vi "Disconnect.vi"(8 "error in (no error)":errorcluster, 11 "PalmSens in":refnum<class "PalmSens.lvclass">) -> (0 "error out":errorcluster, 3 "PalmSens out":refnum<class "PalmSens.lvclass">)   [LabVIEW 2020, in "PalmSens.lvclass"]
uses:
  PalmSens.lvclass
  PalmSens.lvclass/PalmSens.ctl
  C:/Utils/LabVIEWNETSDK - Class/PalmSens/Libraries/PalmSens.Core.Simplified.LabVIEW.dll
  Libraries/PalmSens.Core.Simplified.LabVIEW.dll
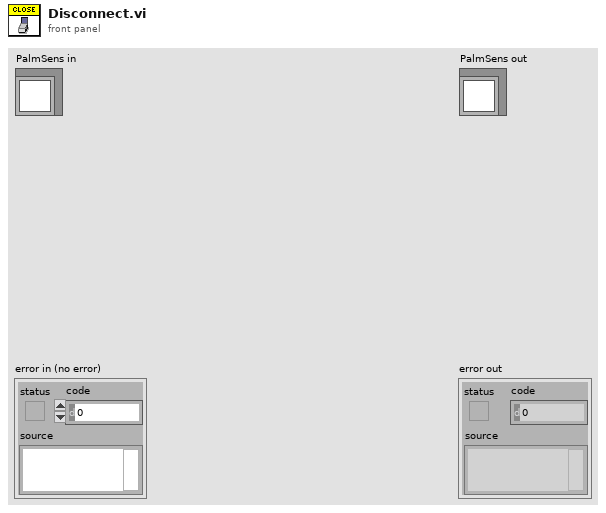
[diagram p1: front panel]
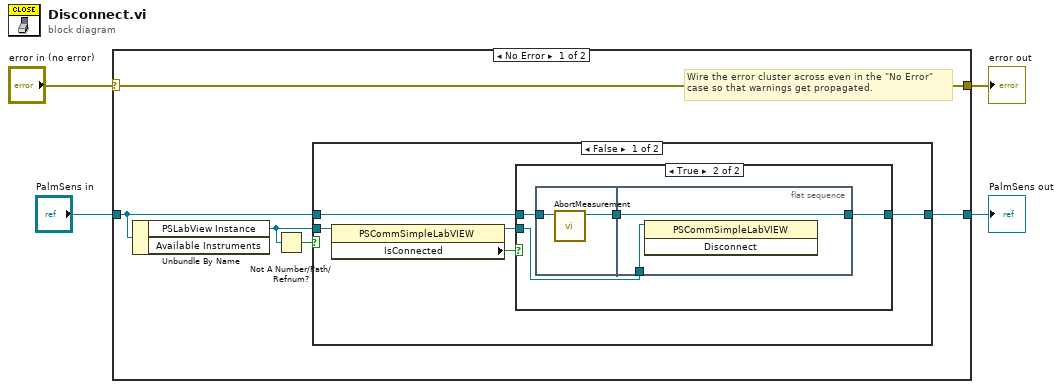
[diagram p0: block diagram]
diagram:
  n1 = case shown="No Error" "error in (no error)" {
    selector: "error in (no error)" -> [w9 w26]
    tunnel: [w9 w26] -> w3
    tunnel: [w5 w25] -> w1
    tunnel: "PalmSens in" -> [w6 w25]
    frame No Error {
      # "Wire the error cluster across even in the \"No Error\"\ncase so that warnings get propagated."
      n2 = Unbundle By Name(w6) -> ("PSLabView Instance"=w7:refnum<k24>)  [unwired: 1 out]
      n3 = Not A Number/Path/Refnum?(number/path/refnum=w7) -> (NaN/Path/Refnum?=w8:bool)
      n4 = case shown="False" w8 {
        tunnel: w7 -> [w14 _]
        tunnel: w6 -> [w11 w24]
        tunnel: [w10 w24] -> w5
        frame False {
          n5 = property class="PSCommSimpleLabVIEW"(reference=w14) -> (reference out=w12:refnum<k24>, "IsConnected"=w13:bool)  [unwired: 1 in, 1 out]
          n6 = case shown="True" w13 {
            tunnel: w12 -> [_ w16]
            tunnel: w11 -> [w15 w19]
            tunnel: [w15 w18] -> w10
            frame False {
            }
            frame True {
              n7 = flat-sequence {
                tunnel: w19 -> [w21]
                tunnel: [w20] -> w17
                tunnel: [w23] -> w18
                tunnel: w17 -> [w23]
                tunnel: w16 -> [w22]
                frame #0 {
                  n8 = call-dynamic "AbortMeasurement.vi"("PalmSens in"=w21) -> ("PalmSens out"=w20:refnum<class "PalmSens.lvclass">)  [unwired: 9 in, 1 out]
                }
                frame #1 {
                  n9 = invoke class="PSCommSimpleLabVIEW" method="Disconnect"(reference=w22) -> ()  [unwired: 2 in, 3 out]
                }
              }
            }
          }
        }
        frame True {
        }
      }
    }
    frame Error {
    }
  }
  "error out" <- w3
  "PalmSens out" <- w1
